vi "Anterior_Posterior_A_Numero.vi"(4 "Limite_Superior":dbl, 7 "Numero":dbl) -> (0 "Cumple_Limite_Superior":bool, 1 "Cumple_Limite_Inferior":bool, 2 "Posterior":dbl, 3 "Anterior":dbl)   [LabVIEW 2019]
doc: "Recibe como parametros un 'numero' y un 'Limite_Superior' de tipo enteros\n\nRetorna 'Anterior' que es la resta de 'numero' - 1.\nRetorna 'Posterior' que es la suma de 'numero' + 1.\nRetorna 'Cumple_Limite_Inferior' si la resta anterior es mayor o igual a cero.\nRetorna 'Cumple_Limite_Superior' si la suma anterior es menor al 'Limite_Superior'."
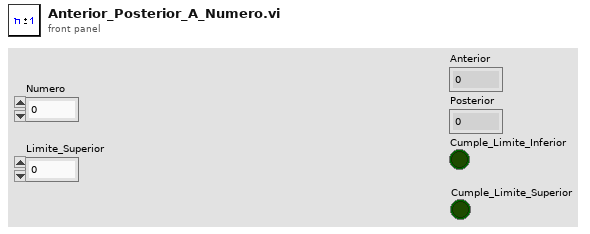
[diagram p1: front panel]
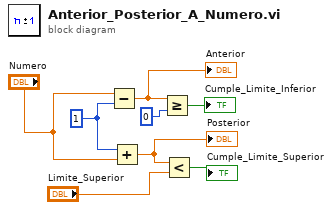
[diagram p0: block diagram]
diagram:
  w6 = 1 ("y")
  n1 = Subtract(x="Numero", y=w6) -> (x-y=w5:dbl)
  "Anterior" <- w5
  n2 = Add(x=w6, y="Numero") -> (x+y=w4:dbl)
  "Posterior" <- w4
  n3 = Greater Or Equal?(x=w5, y=0) -> (x >= y?=→"Cumple_Limite_Inferior":bool)
  n4 = Less?(x=w4, y="Limite_Superior") -> (x < y?=→"Cumple_Limite_Superior":bool)
